vi "74HC153功能测试.vi"(0 "D10":bool, 1 "D11":bool, 2 "D12":bool, 3 "D13":bool, 4 "D20":bool, 5 "D21":bool, 6 "D22":bool, 7 "D23":bool, 8 "S0":bool, 9 "S1":bool, 12 "EN1":bool, 13 "EN2":bool) -> ()   [LabVIEW 2018]
panel:
  in  "结束":bool
  out "Y2":bool
  out "Y1":bool
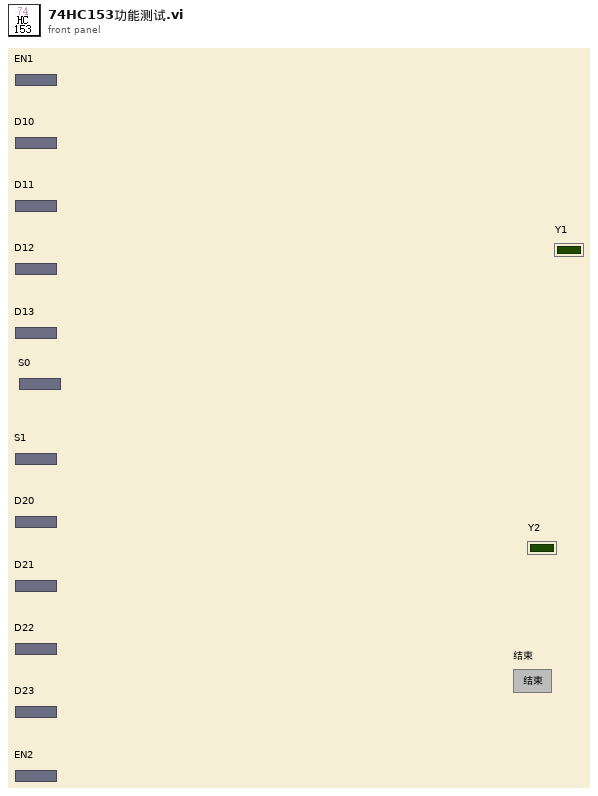
[diagram p1: front panel]
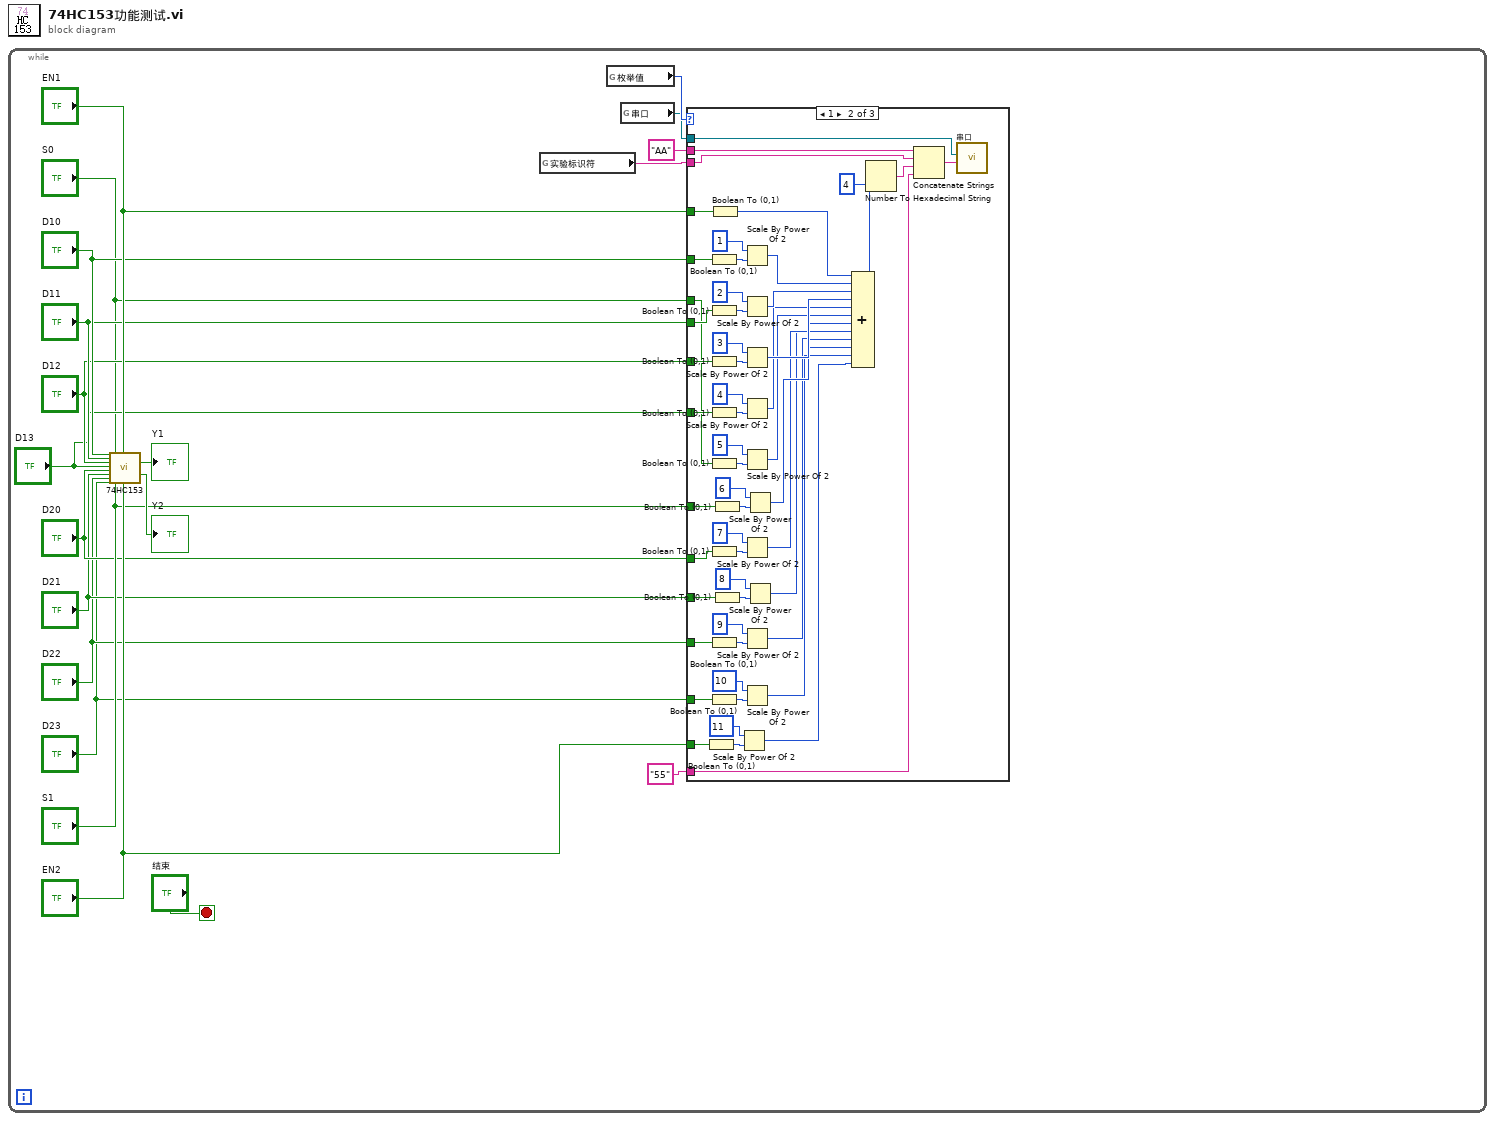
[diagram p0: block diagram]
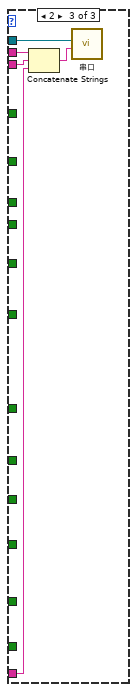
[diagram p3: hidden frame]
diagram:
  n1 = while {
    stop <- "结束" stop-if-true
    n2 = call "74HC153.vi"("D10"="D10", "D11"="D11", "D12"="D12", "D13"="D13", "D20"="D20", "D21"="D21", "D22"="D22", "D23"="D23", "S0"="S0", "S1"="S1", "EN1"="EN1", "EN2"="EN2") -> ("Y1"=→"Y1":bool, "Y2"=→"Y2":bool)  [unwired: 14 in]
    n3 = global read "全局变量.vi" "实验标识符"() -> (w15:string)
    n4 = global read "全局变量.vi" "枚举值"() -> (w17:i8)
    n5 = global read "全局变量.vi" "串口"() -> (w16:refnum<visa-resource-name>)
    n6 = case shown="1" w17 {
      tunnel: w16 -> [_ w69 w77]
      tunnel: w15 -> [_ w68 w78]
      tunnel: "55" -> [_ w67 w75]
      tunnel: "AA" -> [_ w66 w76]
      tunnel: "EN1" -> [_ w32 _]
      tunnel: "EN2" -> [_ w31 _]
      tunnel: "D10" -> [_ w30 _]
      tunnel: "D11" -> [_ w29 _]
      tunnel: "D12" -> [_ w28 _]
      tunnel: "D13" -> [_ w27 _]
      tunnel: "S0" -> [_ w26 _]
      tunnel: "S1" -> [_ w25 _]
      tunnel: "D20" -> [_ w24 _]
      tunnel: "D21" -> [_ w23 _]
      tunnel: "D22" -> [_ w22 _]
      tunnel: "D23" -> [_ w21 _]
      frame 0, Default {
      }
      frame 1 {
        n7 = Boolean To (0,1)(Boolean=w31) -> (0, 1=w40:i16)
        n8 = Boolean To (0,1)(Boolean=w30) -> (0, 1=w71:i16)
        n9 = Boolean To (0,1)(Boolean=w29) -> (0, 1=w61:i16)
        n10 = Boolean To (0,1)(Boolean=w28) -> (0, 1=w59:i16)
        n11 = Boolean To (0,1)(Boolean=w27) -> (0, 1=w57:i16)
        n12 = Boolean To (0,1)(Boolean=w26) -> (0, 1=w55:i16)
        n13 = Boolean To (0,1)(Boolean=w24) -> (0, 1=w48:i16)
        n14 = Boolean To (0,1)(Boolean=w22) -> (0, 1=w44:i16)
        n15 = Boolean To (0,1)(Boolean=w21) -> (0, 1=w42:i16)
        n16 = Boolean To (0,1)(Boolean=w32) -> (0, 1=w73:i16)
        n17 = Boolean To (0,1)(Boolean=w25) -> (0, 1=w50:i16)
        n18 = Boolean To (0,1)(Boolean=w23) -> (0, 1=w46:i16)
        n19 = Scale By Power Of 2(n=11, x=w40) -> (x*2^n=w33:i16)
        n20 = Scale By Power Of 2(n=1, x=w71) -> (x*2^n=w72:i16)
        n21 = Scale By Power Of 2(n=2, x=w61) -> (x*2^n=w62:i16)
        n22 = Scale By Power Of 2(n=3, x=w59) -> (x*2^n=w53:i16)
        n23 = Scale By Power Of 2(n=4, x=w57) -> (x*2^n=w52:i16)
        n24 = Scale By Power Of 2(n=5, x=w55) -> (x*2^n=w51:i16)
        n25 = Scale By Power Of 2(n=7, x=w48) -> (x*2^n=w37:i16)
        n26 = Scale By Power Of 2(n=9, x=w44) -> (x*2^n=w35:i16)
        n27 = Scale By Power Of 2(n=10, x=w42) -> (x*2^n=w34:i16)
        n28 = Scale By Power Of 2(n=6, x=w50) -> (x*2^n=w38:i16)
        n29 = Scale By Power Of 2(n=8, x=w46) -> (x*2^n=w36:i16)
        n30 = Compound Arithmetic op=ADD ("复合运算")(w73, w72, w62, w53, w52, w51, w38, w37, w36, w35, w34, w33) -> (w65:i16)
        n31 = Number To Hexadecimal String(1:4, 2:w65) -> (0:w63:string)
        n32 = Concatenate Strings(w66, w68, w63, w67) -> (w74:string)
        n33 = call "串口.vi"("字符串"=w74, "VISA resource name"=w69) -> ()  [unwired: 10 in]
      }
      frame 2 {
        n34 = Concatenate Strings(w76, w78, w75) -> (w79:string)
        n35 = call "串口.vi"("字符串"=w79, "VISA resource name"=w77) -> ()  [unwired: 10 in]
      }
    }
  }
